vi "write_attributes.vi"(8 "error in (no error)":errorcluster, 10 "attributes":T1, 11 "OrthogonalMatchingPursuitCV in":refnum<class "OrthogonalMatchingPursuitCV.lvclass">) -> (0 "error out":errorcluster, 3 "OrthogonalMatchingPursuitCV out":refnum<class "OrthogonalMatchingPursuitCV.lvclass">)   [LabVIEW 2020, in "OrthogonalMatchingPursuitCV.lvclass"]
uses:
  OrthogonalMatchingPursuitCV.lvclass
  Controls/orthogonal_matching_pursuit_cv_attributes.ctl
  OrthogonalMatchingPursuitCV.lvclass/OrthogonalMatchingPursuitCV.ctl
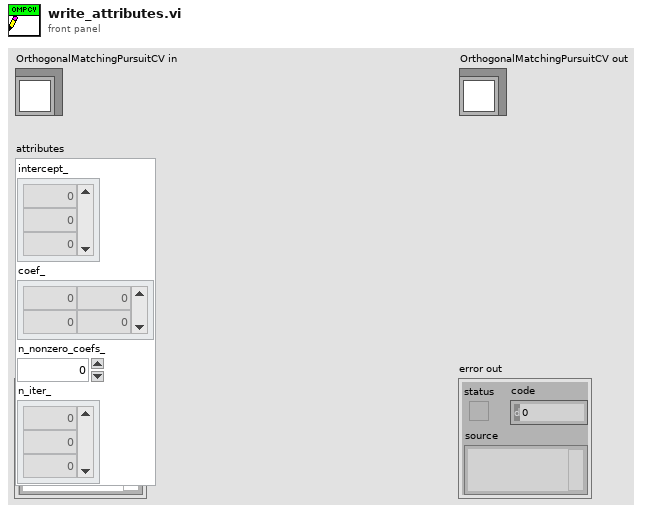
[diagram p1: front panel]
types:
  T1 = typedef "orthogonal_matching_pursuit_cv_attributes.ctl" = cluster{"intercept_":dbl[], "coef_":dbl[][], "n_nonzero_coefs_":dbl, "n_iter_":dbl[]}
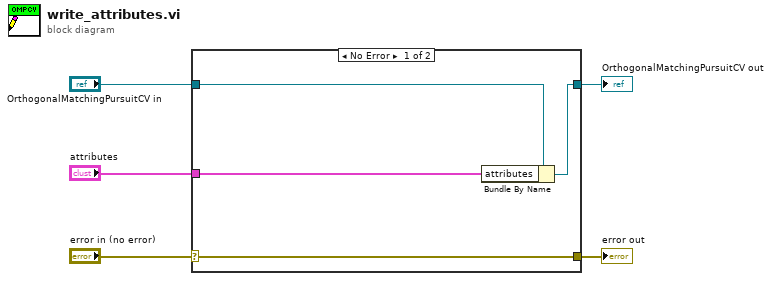
[diagram p0: block diagram]
diagram:
  n1 = case shown="No Error" "error in (no error)" {
    selector: "error in (no error)" -> [w9 w10]
    tunnel: [w9 w10] -> w4
    tunnel: [w7 w11] -> w2
    tunnel: "OrthogonalMatchingPursuitCV in" -> [w8 w11]
    tunnel: "attributes" -> [w6 _]
    frame No Error {
      n2 = Bundle By Name(cluster=w8, "attributes"=w6) -> (w7:refnum<class "OrthogonalMatchingPursuitCV.lvclass">)
    }
    frame Error {
    }
  }
  "error out" <- w4
  "OrthogonalMatchingPursuitCV out" <- w2
